vi "Get rig specific files path.vi"() -> (1 "Rig-specific files folder (string)":string, 3 "Rig-specific files folder":path)   [LabVIEW 2013]
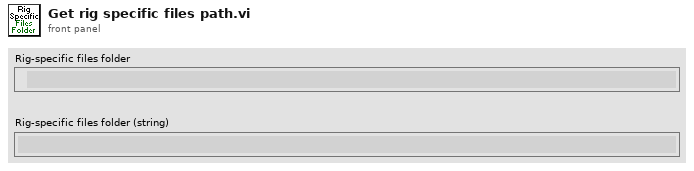
[diagram p1: front panel]
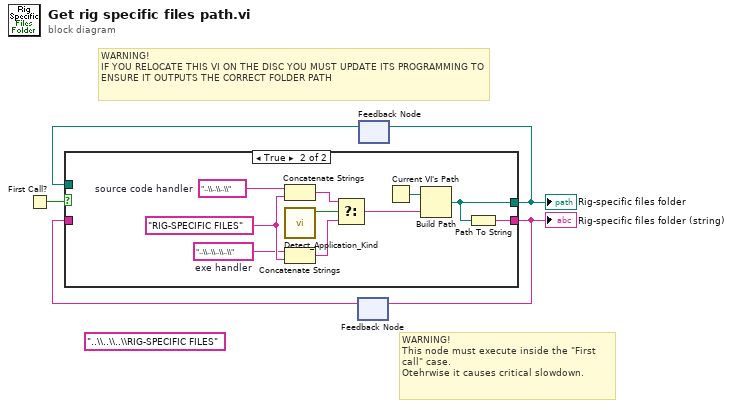
[diagram p0: block diagram]
diagram:
  (unwired) "..\\..\\..\\RIG-SPECIFIC FILES"
  # "WARNING!\nThis node must execute inside the \"First call\" case.\nOtehrwise it causes critical slowdown."
  # "WARNING!\nIF YOU RELOCATE THIS VI ON THE DISC YOU MUST UPDATE ITS PROGRAMMING TO ENSURE IT OUTPUTS THE CORRECT FOLDER PATH"
  n1 = First Call?() -> (First Call?: T/F=w3:bool)
  n2 = feedback #1() -> (w1:string)  [unwired: 1 in]
  n3 = feedback #2() -> (w5:path)  [unwired: 1 in]
  n4 = case shown="True" w3 {
    tunnel: [w7 w16] -> w4
    tunnel: w5 -> [w7 _]
    tunnel: [w6 w15] -> w2
    tunnel: w1 -> [w6 _]
    frame False {
    }
    frame True {
      w14 = "RIG-SPECIFIC FILES"
      w12 = "..\\..\\..\\"  # source code handler
      w11 = "..\\..\\..\\..\\"  # exe handler
      n5 = Concatenate Strings(w12, w14) -> (w13:string)
      n6 = call "Detect_Application_Kind.vi"() -> ("Development System"=w9:bool)  [unwired: 9 in, 2 out]
      n7 = Concatenate Strings(w11, w14) -> (w10:string)
      n8 = Select(t=w13, s=w9, f=w10) -> (s? t:f=w8:string)
      n9 = Current VI's Path() -> (path=w17:path)
      n10 = Build Path(base path=w17, name or relative path=w8) -> (appended path=w16:path)
      n11 = Path To String(path=w16) -> (string=w15:string)
    }
  }
  "Rig-specific files folder" <- w4
  "Rig-specific files folder (string)" <- w2
  n12 = feedback-in #1(w2) -> ()
  n13 = feedback-in #2(w4) -> ()
